vi "Build Scan Graph.vi"(8 "error in":errorcluster, 11 "Scan Driver in":refnum<class "Scan Driver.lvclass">) -> (0 "error out":errorcluster, 1 "Secondary Graph":T1, 2 "Primary Graph":T1=[{"point array"=[{"x"=401.0007, "y"=8.19568e-08}, {"x"=401.9996, "y"=4.65664e-09}, {"x"=403.0005, "y"=8.38195e-08}, {"x"=403.9992, "y"=-1.67639e-07}, {"x"=404.9998, "y"=-6.70557e-08}, {"x"=406.0002, "y"=-2.88712e-07}, {"x"=407.00059999999996, "y"=2.1793e-07}, {"x"=408.0007, "y"=3.72531e-08}, {"x"=409.0008, "y"=-6.89183e-08}, {"x"=410.0006, "y"=-1.49013e-08}]}], 3 "Scan Driver out":refnum<class "Scan Driver.lvclass">)   [LabVIEW 2009, in "Scan Driver.lvclass"]
doc: "Build and return the updated scan graph from the data store."
uses:
  Scan Driver.lvclass
  Scan Graph.ctl
  Scan Driver.lvclass/Scan Driver.ctl
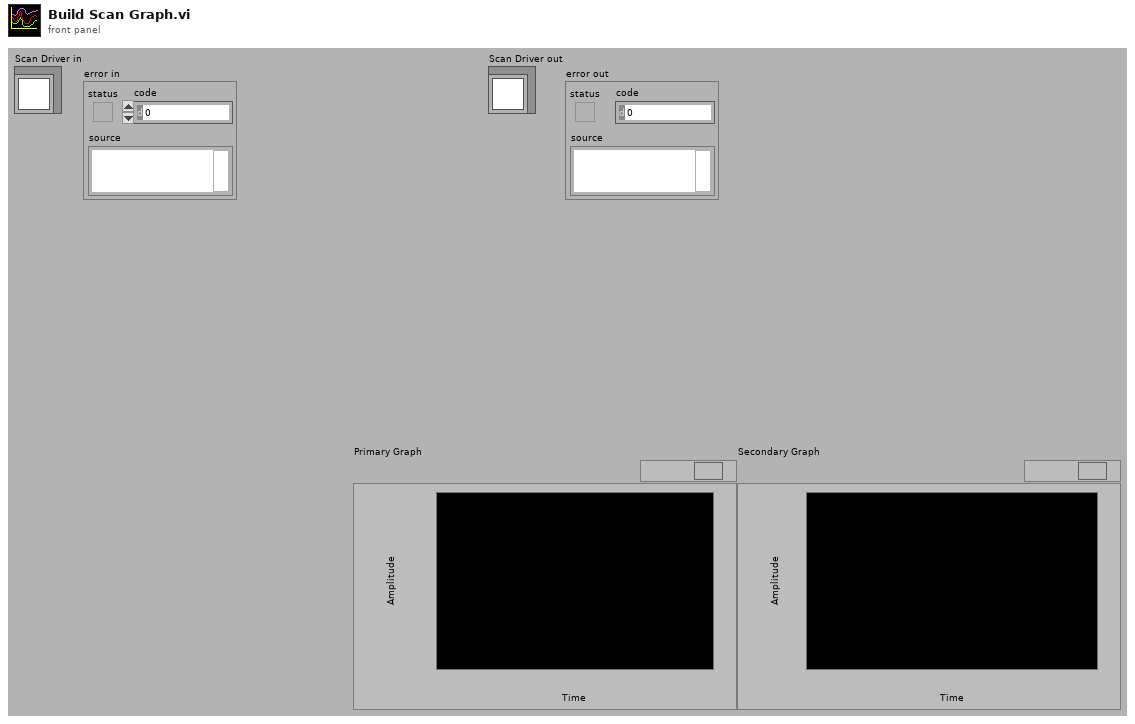
[diagram p1: front panel]
types:
  T1 = typedef "Scan Driver.lvclass/Scan Graph.ctl" = cluster{"point array":cluster{"x":dbl, "y":dbl}[]}[]
  T2 = cluster{"Data Column Headings":string[], "Primary Plot Labels":string[], "Secondary Plot Labels":string[], "Tag":string, "Y-axis":string, "Total # Columns (incl. X-var)":dbl, "Index of first Secondary\nColumn (from 0)":dbl, "# Secondary Columns":dbl, "# Data Columns (deprecated)":dbl, "# Data Columns":dbl}
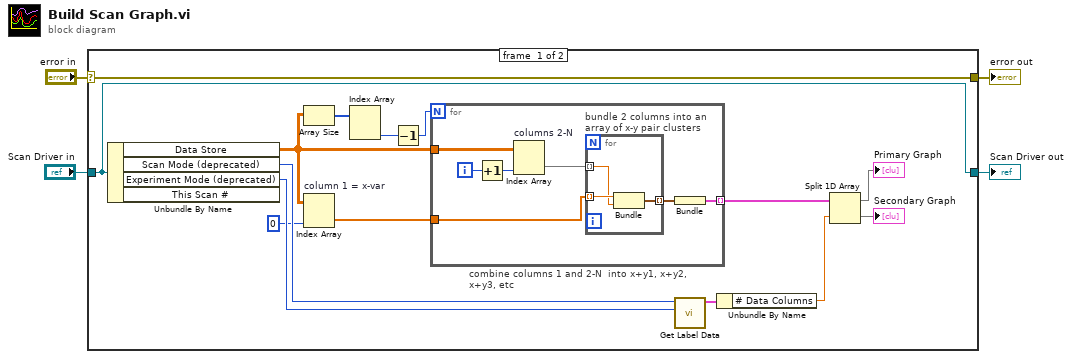
[diagram p0: block diagram]
diagram:
  n1 = case shown="No Error" "error in" {
    selector: "error in" -> [w19 w31]
    tunnel: [w19 w31] -> w3
    tunnel: "Scan Driver in" -> [w6 w30]
    tunnel: [w6 w30] -> w1
    frame #0 {
      n2 = Unbundle By Name(w6) -> ("Data Store"=w9:dbl[][], "Scan Mode (deprecated)"=w18:u8, "Experiment Mode (deprecated)"=w14:u8)  [unwired: 1 out]
      n3 = Array Size(array=w9) -> (size(s)=w13:i32[])
      n4 = Index Array "column 1 = x-var"(array=w9, index (col)=0) -> (element=w15:dbl[])  [unwired: 1 in]
      n5 = Index Array(array=w13) -> (element #2=w5:i32)  [unwired: 2 in, 1 out]
      n6 = Decrement(x=w5) -> (x-1=w10:i32)
      n7 = for "combine columns 1 and 2-N  into x+y1, x+y2, x+y3, etc" {
        N: w10 -> [_]
        tunnel: w15 -> [w22]
        tunnel: w9 -> [w26]
        tunnel: [w21] -> w7 mode=indexing
        i -> [w25]
        n8 = Increment(x=w25) -> (x+1=w24:i32)
        n9 = Index Array "columns 2-N"(array=w26, index (col)=w24) -> (element=w23:dbl[])  [unwired: 1 in]
        n10 = for "bundle 2 columns into an\narray of x-y pair clusters" {
          tunnel: w23 -> [w28] mode=indexing
          tunnel: w22 -> [w29] mode=indexing
          tunnel: [w27] -> w20 mode=indexing
          n11 = Bundle(w29, w28) -> (w27:cluster{dbl, dbl})  [unwired: 1 out]
        }
        n12 = Bundle(w20) -> (w21:cluster{cluster{dbl, dbl}[]})  [unwired: 1 in]
      }
      n13 = call "Get Label Data.vi"("expmode"=w14, "scanmode"=w18) -> ("data"=w12:T2)  [unwired: 9 out]
      n14 = Unbundle By Name(w12) -> ("# Data Columns"=w11:dbl)
      n15 = Split 1D Array(array=w7, index=w11) -> (first subarray=→"Primary Graph":cluster{cluster{dbl, dbl}[]}[], second subarray=→"Secondary Graph":cluster{cluster{dbl, dbl}[]}[])
    }
    frame #1 {
    }
  }
  "error out" <- w3
  "Scan Driver out" <- w1
